vi "Creator Alias.vi"(11 "TEMPLATE jettl in":refnum<class "TEMPLATE Actor.lvclass">) -> (2 "Creator Alias":string)   [LabVIEW 2021, in "_Template.lvlib" / "Templates.lvlib" / "TEMPLATE Actor.lvlib" / "TEMPLATE Actor.lvclass"]
uses:
  TEMPLATE Actor.lvclass
  jettl/jettl/jettl/jettl.lvclass
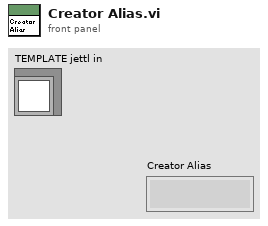
[diagram p1: front panel]
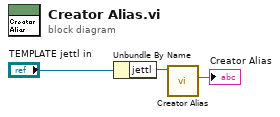
[diagram p0: block diagram]
diagram:
  n1 = Unbundle By Name("TEMPLATE jettl in") -> ("jettl"=w1:refnum<class "jettl.lvclass">)
  n2 = call-dynamic "Creator Alias.vi"("jettl in"=w1) -> ("Creator Alias"=→"Creator Alias":string)  [unwired: 10 in]
